vi "题目三.vi"() -> ()   [LabVIEW 2017]
panel:
  in  "停止":bool
  out "温度计 2":dbl(slide) scale=0.0..260.0
  in  "温度单位":bool
  out "温度":string
  # "°C"
  # "°F"
  # "°C"
  # "°F"
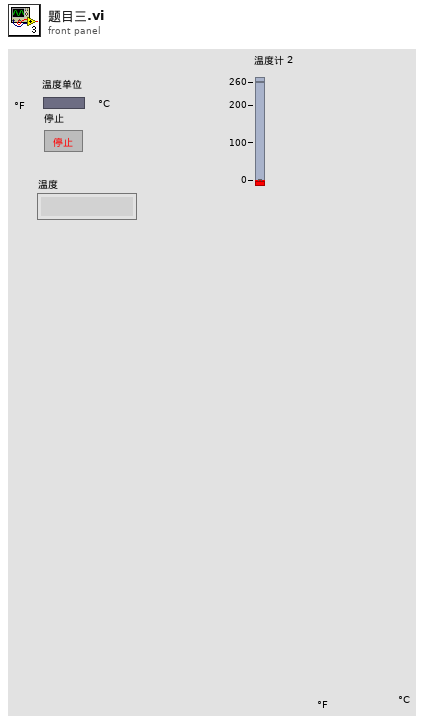
[diagram p1: front panel]
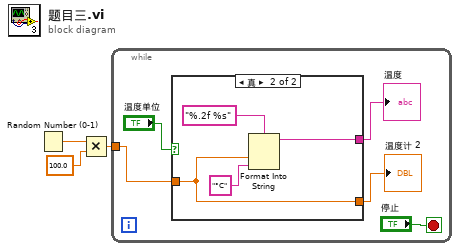
[diagram p0: block diagram]
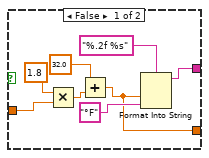
[diagram p2: hidden frame]
diagram:
  n1 = Random Number (0-1)() -> (number: 0 to 1=w3:dbl)
  n2 = Multiply(x=w3, y=100.0) -> (x*y=w1:dbl)
  n3 = while {
    tunnel: w1 -> [w8]
    stop <- "停止" stop-if-true
    n4 = case shown="真" "温度单位" {
      tunnel: w8 -> [w14 w17]
      tunnel: [w10 w19] -> w6
      tunnel: [w9 w17] -> w5
      frame False {
        n5 = Multiply(x=1.8, y=w14) -> (x*y=w12:dbl)
        n6 = Add(x=32.0, y=w12) -> (x+y=w9:dbl)
        n7 = Format Into String(format string="%.2f %s" ("格式字符串"), w9, "°F") -> (resulting string=w10:string)  [unwired: 2 in, 1 out]
      }
      frame True {
        n8 = Format Into String(format string="%.2f %s" ("格式字符串"), w17, "°C") -> (resulting string=w19:string)  [unwired: 2 in, 1 out]
      }
    }
    "温度" <- w6
    "温度计 2" <- w5
  }
